vi "Register Self.vi"(5 "Ownwer":refnum<class "UniqueName.lvclass">, 7 "Module Name":string, 10 "error in (no error)":errorcluster, 11 "vi reference in":refnum<vi>) -> (2 "error out":errorcluster, 3 "vi reference out":refnum<vi>)   [LabVIEW 2014, in "ConfigurableQMH.lvlib"]
uses:
  ConfigurableQMH.lvlib
  <vilib>/LabVIEW Open Source Project/Unicity/UniqueName/UniqueNameClass/UniqueName.lvclass
  <vilib>/LabVIEW Open Source Project/Unicity/UniqueName/Registry/NameRegistry.lvclass
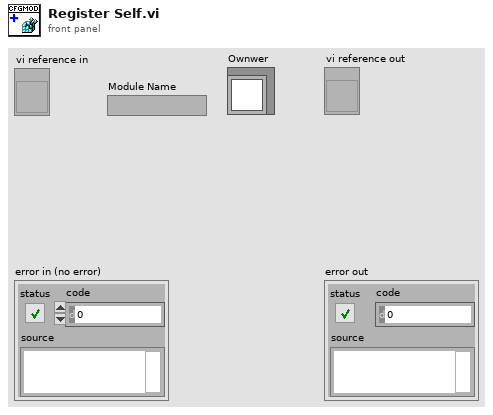
[diagram p1: front panel]
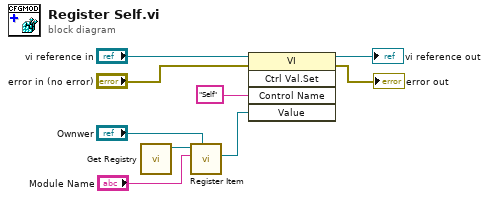
[diagram p0: block diagram]
diagram:
  n1 = call "Get Registry.vi"() -> ("Registry"=w6:refnum<data-value>)  [unwired: 11 in]
  n2 = call <vilib>:"Register Item.vi"("Owner"="Ownwer", "New Object Name"="Module Name", "Registry in"=w6) -> ("New Node"=w7:refnum<class "UniqueName.lvclass">)  [unwired: 6 in, 2 out]
  n3 = invoke class="VI" method="Ctrl Val.Set"(reference="vi reference in", error in="error in (no error)", "Control Name"="Self", "Value"=w7) -> (reference out=→"vi reference out":refnum<vi>, error out=→"error out":errorcluster)  [unwired: 1 in, 3 out]
